vi "LoadParameters.vi"(8 "error in (no error)":errorcluster, 9 "Command line args":string[](array[string]), 11 "CDependencyInspection in":refnum<class "CDependencyInspection.lvclass">) -> (0 "error out":errorcluster, 3 "CDependencyInspection out":refnum<class "CDependencyInspection.lvclass">)   [LabVIEW 2020, in "DependencyInspection.lvlib" / "CDependencyInspection.lvclass"]
uses:
  CDependencyInspection.lvclass
  CommonHelpers/CommonHelpers.lvlib
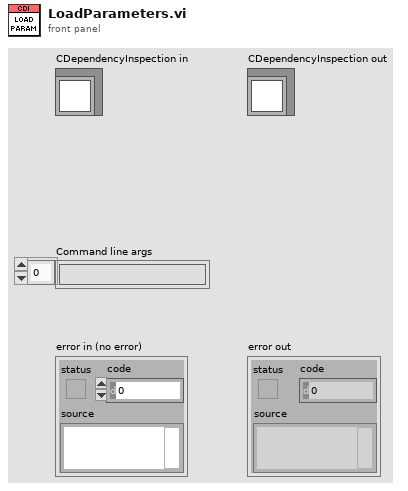
[diagram p1: front panel]
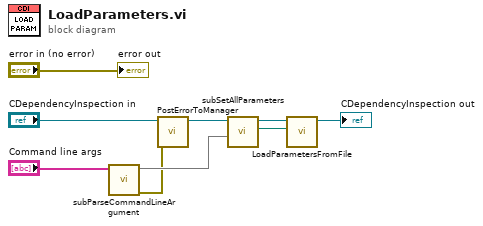
[diagram p0: block diagram]
diagram:
  n1 = call "subParseCommandLineArgument.vi"("Command line args"="Command line args") -> ("error out"=w1:errorcluster, "Parameters"=w5:map{string, string})  [unwired: 9 in]
  n2 = call-dynamic "PostErrorToManager.vi"("error in (no error)"=w1, "CDependencyInspection in"="CDependencyInspection in") -> ("CDependencyInspection out"=w2:refnum<class "CDependencyInspection.lvclass">)  [unwired: 8 in, 1 out]
  n3 = call "subSetAllParameters.vi"("Parameters"=w5, "CDependencyInspection in"=w2) -> ("Config file path"=w4:path, "CDependencyInspection out"=w9:refnum<class "CDependencyInspection.lvclass">)  [unwired: 7 in, 1 out]
  n4 = call-dynamic "LoadParametersFromFile.vi"("Config file path"=w4, "CDependencyInspection in"=w9) -> ("CDependencyInspection out"=→"CDependencyInspection out":refnum<class "CDependencyInspection.lvclass">)  [unwired: 8 in, 1 out]
  "error out" <- "error in (no error)"
